vi "Initiate Acquisition.vi"(8 "error in (no error)":errorcluster {"code" format="%.0x"}, 11 "VISA Resource Name":refnum<visa-resource-name>) -> (0 "error out":errorcluster {"code" format="%.0x"}, 3 "VISA Resource Name Out":refnum<visa-resource-name>)   [LabVIEW 2011, in "Agilent 546XX Series.lvlib"]
doc: "This VI initiates an acquisition on the channels that you enable with the ag546xx Configure Channel VI. It then waits for the acquisition to complete, and returns the waveform for the channel you specify. You call the ag546xx Fetch Waveform VI to obtain the waveforms for each of the remaining enabled channels without initiating another acquisition.\n\nNotes:\n\n(1) After this VI executes, each element in the Waveform Array is either a voltage or a value indicating that the oscilloscope could not sample a voltage."
uses:
  Agilent 546XX Series.lvlib
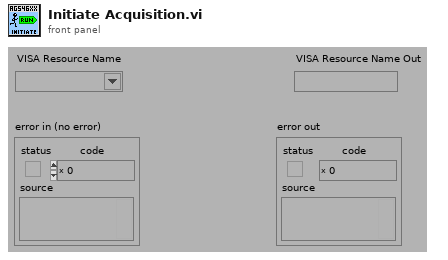
[diagram p1: front panel]
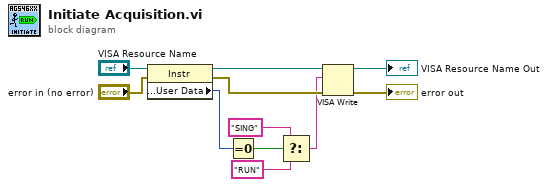
[diagram p0: block diagram]
diagram:
  n1 = property class="Instr"(reference="VISA Resource Name", error in="error in (no error)") -> (reference out=w5:refnum<visa-resource-name>, error out=w4:errorcluster, "General Settings:User Data"=w8:u32)
  n2 = Equal To 0?(x=w8) -> (x = 0?=w9:bool)
  n3 = Select(t="SING", s=w9, f="RUN") -> (s? t:f=w1:string)
  n4 = VISA Write(VISA resource name=w5, write buffer=w1, error in (no error)=w4) -> (VISA resource name out=→"VISA Resource Name Out":refnum<visa-resource-name>, error out=→"error out":errorcluster)  [unwired: 1 out]
